vi "Plot Measures.vi"(7 "Text Color (red)":u32(colorbox)=16711680, 8 "error in":errorcluster, 10 "Measurements":T1(array[cluster]), 11 "Image In":T2) -> (0 "error out":errorcluster, 3 "Image Out":T2)   [LabVIEW 2012, in "Visual Analyser.lvlib"]
uses:
  Visual Analyser.lvlib
  <vilib>/vision/Image Controls.llb/IMAQ Image.ctl
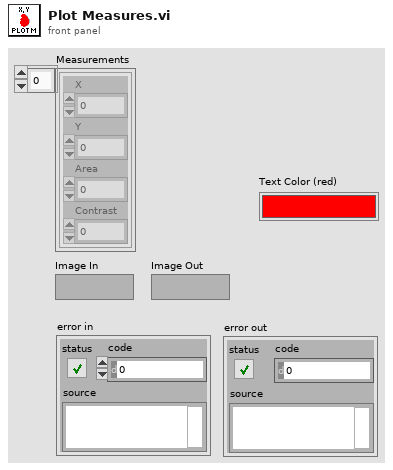
[diagram p1: front panel]
types:
  T1 = cluster{"X":dbl, "Y":dbl, "Area":dbl, "Contrast":dbl}[]
  T2 = typedef "IMAQ Image.ctl" = refnum<image>
  T3 = cluster{"Desired Font (Application)":enum16{"User-specified Font", "Application Font", "System Font", "Dialog Font"}, "[User-specified Font]":cluster{"Font Name":string, "Size":i16, "Strikeout?":bool, "Italic?":bool, "Underline?":bool, "Outline?":bool, "Shadow?":bool, "Bold?":bool, "Rotation Angle":dbl}, "Horizontal Alignment":i16, "Vertical Alignment":i16}
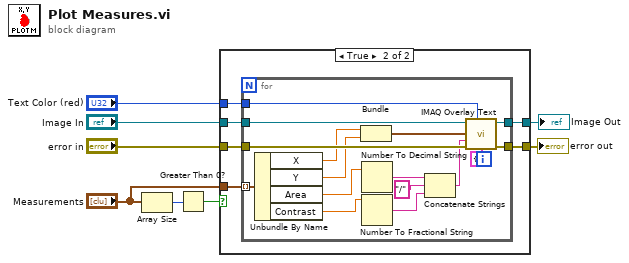
[diagram p0: block diagram]
diagram:
  n1 = Array Size(array="Measurements") -> (size(s)=w2:i32)
  n2 = Greater Than 0?(x=w2) -> (x > 0?=w3:bool)
  n3 = case shown="True" w3 {
    tunnel: [w9 w16] -> w8
    tunnel: "Text Color (red)" -> [_ w15]
    tunnel: "Image In" -> [w10 w14]
    tunnel: [w10 w13] -> w5
    tunnel: "error in" -> [w9 w12]
    tunnel: "Measurements" -> [_ w11]
    frame False {
    }
    frame True {
      n4 = for {
        tunnel: w12 -> [w26]
        tunnel: [w32] -> w16
        tunnel: [w31] -> w13
        tunnel: w14 -> [w30]
        tunnel: w15 -> [w27]
        tunnel: w11 -> [w25] mode=indexing
        n5 = Unbundle By Name(w25) -> ("X"=w24:dbl, "Y"=w23:dbl, "Area"=w22:dbl, "Contrast"=w21:dbl)
        n6 = Bundle("X"=w24, "Y"=w23) -> (w29:cluster{"X":dbl, "Y":dbl})  [unwired: 1 out]
        n7 = Number To Decimal String(number=w22) -> (decimal integer string=w20:string)  [unwired: 1 out]
        n8 = Number To Fractional String(number=w21) -> (F-format string=w19:string)  [unwired: 3 in]
        n9 = Concatenate Strings(w20, "/" ("string"), w19) -> (w17:string)
        n10 = call "IMAQ Overlay Text"("Text Color (black)"=w27, "Font, Size & Style"=T3 {"Desired Font (Application)"=enum."Application Font", "[User-specified Font]"={"Font Name"="", "Size"=12, "Strikeout?"=FALSE, "Italic?"=FALSE, "Underline?"=FALSE, "Outline?"=FALSE, "Shadow?"=FALSE, "Bold?"=FALSE, "Rotation Angle"=0.0}, "Horizontal Alignment"=0, "Vertical Alignment"=0}, "error in (no error)"=w26, "String"=w17, "Origin"=w29, "Image"=w30) -> ("error out"=w32:errorcluster, "Image Out"=w31:T2)  [unwired: 2 in, 2 out]
      }
    }
  }
  "error out" <- w8
  "Image Out" <- w5
